vi "OpenTypeDef-RunTime.vi"(6 "Mouse Position":T1, 7 "User VI Ref":refnum<vi>, 8 "Is Multi-select?":bool, 9 "Remaining Items":refnum<vi>[](array[refnum]), 10 "Affected Items":T8, 11 "Menu Refnum":refnum<k9>) -> (3 "Menu Items To Add":T2[](array[typedef]))   [LabVIEW 2020]
doc: "This VI is part of a plug-in for modifying the LabVIEW shortcut menus. This is the builder VI which is called when the shortcut menu is built. It tells LabVIEW which shortcut menu items to add to the menu."
uses:
  <resource>/plugins/PopupMenus/support/Checkmark Status.ctl
  <resource>/plugins/PopupMenus/support/Relative Position.ctl
  <resource>/plugins/PopupMenus/support/Position In Menu.ctl
  <resource>/plugins/PopupMenus/support/Transaction Control.ctl
  <resource>/plugins/PopupMenus/support/Shortcut Menu Item Definition.ctl
  <resource>/plugins/PopupMenus/support/Enabled Menu Item Status.ctl
  <vilib>/Utility/Data Type/Type Definitions/Data Type.ctl
  <vilib>/Utility/Data Type/NI_Data Type.lvlib
  OpenTypeDef-RunTime.ctl
  <vilib>/Utility/miscctls.llb/LVPositionTypeDef.ctl
panel:
  # "Rules a popup plug-in must follow:\n* This VI's file name must match the file name of the LLB -- only the file extensions should be different.\n* This VI must have debugging disabled or it will be ignored as a plug-in.\n* For all menu items, \"tag suffix + file name of this VI\" must be less than 240 characters.\n* You can disconnect the \"Affected Items\" from the typedef to make the plug-in load faster. The typedef is only there to assist you in keeping this VI and the execution VI using to the same type.\n* All controls on this panel except \"Affected Items\" are locked to prevent accidental edits. Do not change the types or the names of controls other than the elements inside the \"Affected Items\" cluster.\n* See Context Help for more information on the individual controls."
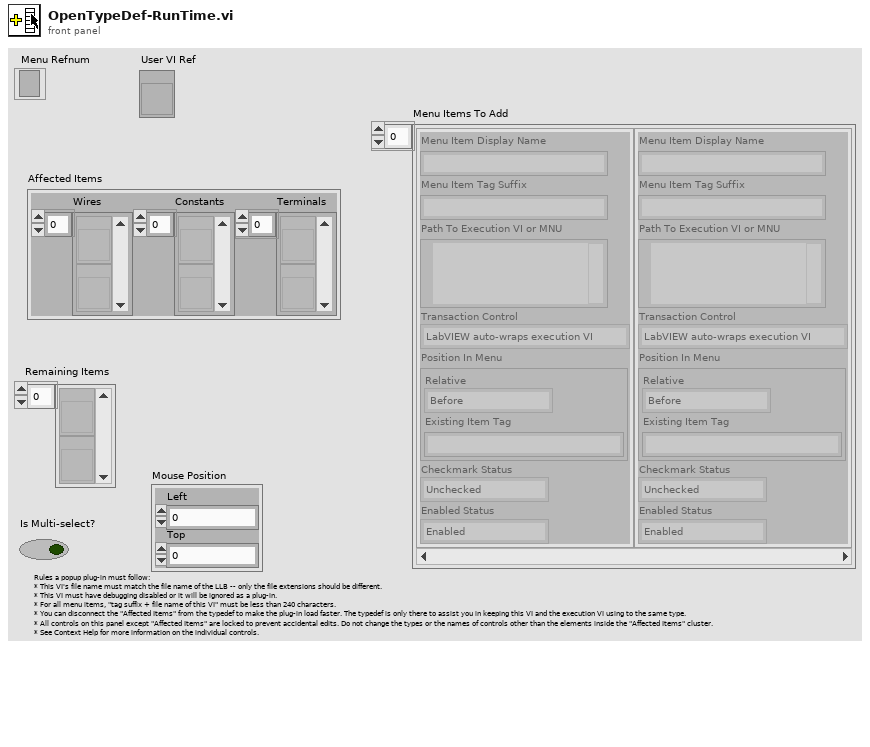
[diagram p1: front panel]
types:
  T1 = typedef "LVPositionTypeDef.ctl" = cluster{"Left":i32, "Top":i32}
  T2 = typedef "Shortcut Menu Item Definition.ctl" = cluster{"Menu Item Display Name":string, "Menu Item Tag Suffix":string, "Path To Execution VI or MNU":path, "Transaction Control":T3, "Position In Menu":T4, "Checkmark Status":T6, "Enabled Status":T7}
  T3 = typedef "Transaction Control.ctl" = enum8{"LabVIEW auto-wraps execution VI", "Execution VI will define if needed"}
  T4 = typedef "Position In Menu.ctl" = cluster{"Relative":T5, "Existing Item Tag":string}
  T5 = typedef "Relative Position.ctl" = enum8{"Before", "Instead of", "After", "Into Submenu"}
  T6 = typedef "Checkmark Status.ctl" = enum8{"Unchecked", "Checked"}
  T7 = typedef "Enabled Menu Item Status.ctl" = enum8{"Enabled", "Disabled"}
  T8 = typedef "OpenTypeDef-RunTime.ctl" = cluster{"Wires":refnum<vi>[], "Constants":refnum<vi>[], "Terminals":refnum<vi>[]}
  T9 = typedef "NI_Data Type.lvlib/Data Type.ctl" = enum8{"Invalid Type", "Void", "I8", "I16", "I32", "I64", "U8", "U16", "U32", "U64", "Single Float", "Double Float", "Extended Float", "Single Complex", "Double Complex", "Extended Complex", "Enum U8", "Enum U16", "Enum U32", "Enum U64", "Single Float With Unit", "Double Float With Unit", "Extended Float With Unit", "Single Complex with Unit", "Double Complex with Unit", "Extended Complex with Unit", "Boolean", "String", "Path", "Picture", "Tag", "Array", "Cluster", "Variant", "LV Variant", "Waveform", "Timestamp", "Digital Waveform", "Digital Data", "ExpressData", "Refnum", "External Data", "VI", "Poly VI", "LabVIEW Class Instance", "Fixed Point", "Set Collection", "Map Collection"}
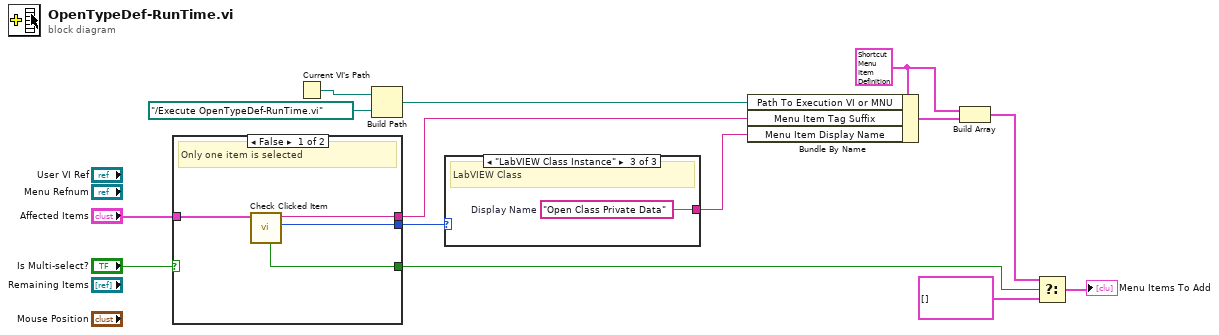
[diagram p0: block diagram]
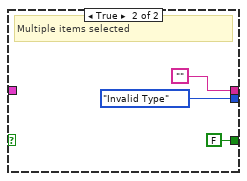
[diagram p2: hidden frame]
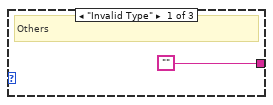
[diagram p3: hidden frame]
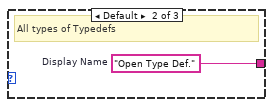
[diagram p4: hidden frame]
diagram:
  w9 = T2 {"Menu Item Display Name"="", "Menu Item Tag Suffix"="", "Path To Execution VI or MNU"=path "", "Transaction Control"=enum."LabVIEW auto-wraps execution VI", "Position In Menu"={"Relative"=enum."Before", "Existing Item Tag"=""}, "Checkmark Status"=enum."Unchecked", "Enabled Status"=enum."Enabled"} ("Cluster")
  n1 = case shown="False" "Is Multi-select?" {
    tunnel: [w17 FALSE ("Typedef/Class Data?")] -> w14
    tunnel: [w15 ""] -> w3
    tunnel: [w16 Data_Type."Invalid Type" ("Type")] -> w2
    tunnel: "Affected Items" -> [w18 _]
    frame False {
      # "Only one item is selected"
      n2 = call "Check Clicked Item.vi"("Affected Items"=w18) -> ("Type"=w16:T9, "Type Definition/Class Path"=w15:string, "Typedef/Class Data?"=w17:bool)  [unwired: 6 in, 1 out]
    }
    frame True {
      # "Multiple items selected"
    }
  }
  n3 = Current VI's Path() -> (path=w11:path)
  n4 = Build Path(base path=w11, name or relative path=path "../Execute OpenTypeDef-RunTime.vi" ("execute path")) -> (appended path=w10:path)
  n5 = case shown="\"LabVIEW Class Instance\"" w2 {
    tunnel: ["" w23 w24] -> w8
    frame "Invalid Type" {
      # "Others"
    }
    frame Default {
      w23 = "Open Type Def."  # Display Name
      # "All types of Typedefs"
    }
    frame "LabVIEW Class Instance" {
      w24 = "Open Class Private Data"  # Display Name
      # "LabVIEW Class"
    }
  }
  n6 = Bundle By Name(cluster=w9, "Path To Execution VI or MNU"=w10, "Menu Item Tag Suffix"=w3, "Menu Item Display Name"=w8) -> (w12:T2)
  n7 = Build Array(w9, w12) -> (w6:T2[])
  n8 = Select(t=w6, s=w14, f=T2[] []) -> (s? t:f=→"Menu Items To Add":T2[])
